vi "Ctor.vi"(5 "SinkType":refnum<class>, 7 "SourceType":refnum<class>, 8 "error in (no error)":errorcluster, 9 "SinkSetter":string, 10 "SourceGetter":string, 11 "PropertyBinder":refnum<class "PropertyBinder.lvclass">) -> (0 "error out":errorcluster, 3 "PropertyBinder":refnum<class "PropertyBinder.lvclass">)   [LabVIEW 2023, in "PropertyBinder.lvclass"]
uses:
  PropertyBinder.lvclass
  ClassReflector/AccessorTypeEnum.ctl
  PropertyBinder.lvclass/PropertyBinder.ctl
  ClassReflector/ClassReflector.lvclass
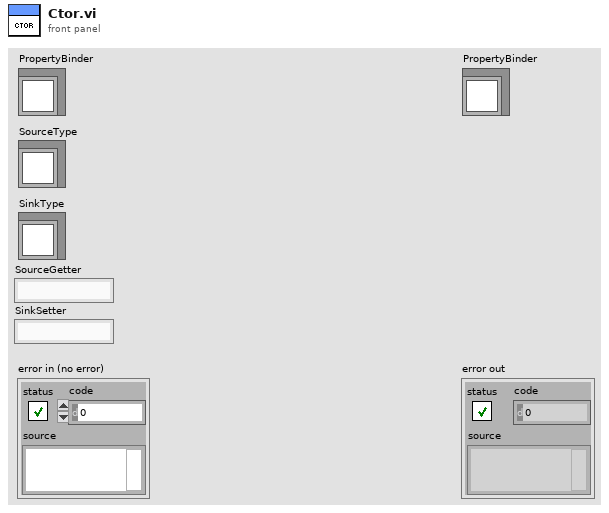
[diagram p1: front panel]
types:
  T1 = typedef "ClassReflector.lvclass/AccessorTypeEnum.ctl" = enum16{"Getter", "Setter"}
  T2 = typedef "ClassReflector.lvclass/AccessorInfoCluster.ctl" = cluster{"VI":refnum<vi>, "ClassInTerm":refnum<vi>, "ClassOutTerm":refnum<vi>, "PropertyTerm":refnum<vi>, "Enum":T1, "QualifiedVIName":string}
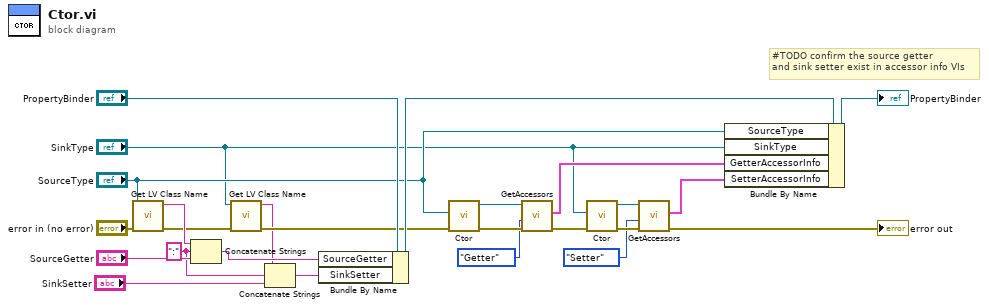
[diagram p0: block diagram]
diagram:
  w7 = ":" ("string")
  # "#TODO confirm the source getter\nand sink setter exist in accessor info VIs"
  n1 = call <vilib>:"Get LV Class Name.vi"("error in (no error)"="error in (no error)", "object"="SourceType") -> ("error out"=w5:errorcluster, "class name"=w9:string)  [unwired: 8 in]
  n2 = Concatenate Strings(w9, w7, "SourceGetter") -> (w8:string)
  n3 = call <vilib>:"Get LV Class Name.vi"("error in (no error)"=w5, "object"="SinkType") -> ("error out"=w4:errorcluster, "class name"=w2:string)  [unwired: 8 in]
  n4 = Concatenate Strings(w2, w7, "SinkSetter") -> (w1:string)
  n5 = Bundle By Name(cluster="PropertyBinder", "SourceGetter"=w8, "SinkSetter"=w1) -> (w14:refnum<class "PropertyBinder.lvclass">)
  n6 = call "Ctor.vi"("error in (no error)"=w4, "Object"="SourceType") -> ("error out"=w24:errorcluster, "ClassReflector out"=w23:refnum<class "ClassReflector.lvclass">)  [unwired: 8 in]
  n7 = call "GetAccessors.vi"("error in (no error)"=w24, "AccessorType"=AccessorTypeEnum."Getter", "ClassReflector in"=w23) -> ("error out"=w22:errorcluster, "GetterAccessorInfo"=w16:T2[])  [unwired: 6 in, 1 out]
  n8 = call "Ctor.vi"("error in (no error)"=w22, "Object"="SinkType") -> ("error out"=w21:errorcluster, "ClassReflector out"=w20:refnum<class "ClassReflector.lvclass">)  [unwired: 8 in]
  n9 = call "GetAccessors.vi"("error in (no error)"=w21, "AccessorType"=AccessorTypeEnum."Setter", "ClassReflector in"=w20) -> ("error out"=→"error out":errorcluster, "GetterAccessorInfo"=w15:T2[])  [unwired: 6 in, 1 out]
  n10 = Bundle By Name(cluster=w14, "SourceType"="SourceType", "SinkType"="SinkType", "GetterAccessorInfo"=w16, "SetterAccessorInfo"=w15) -> (→"PropertyBinder":refnum<class "PropertyBinder.lvclass">)
